vi "Seq Dialog Send LIN Message for inalfa SCU.vi"(8 "Segment Data":T3) -> (0 "Step Hisitory":string[](array[string]), 2 "Segment Data 2":T3)   [LabVIEW 2018]
uses:
  type defs/Sequence Info.ctl
  03.Inalfa LIN/LIN sequence for self SCU.ctl
  03.Inalfa LIN/LIN show Tags.ctl
  03.Inalfa LIN/LIN show messages.ctl
  <vilib>/Utility/error.llb/whitespace.ctl
panel:
  in  "Description":string
  in  "Tx2 2":u8[](array[numeric]) caption="Tx" format="%02x"
  in  "Checksunshade 2":bool=TRUE
  in  "Checkgalss 2":bool=TRUE
  in  "Sunshade Position 2":u16
  in  "Glass Position 2":u16
  in  "Rx 2":u8[](array[numeric]) format="%02x"
  in  "Tx 2":u8[](array[numeric]) format="%02x"
  in  "Slide Cycles 3":u16
  in  "Vent Cycles 3":u16
  in  "Slide Cycles 2":u16
  in  "Vent Cycles 2":u16
  out "LIN show Tags":T1
  in  "Vent Cycles":u16
  in  "Slide Cycles":u16
  in  "String":string
  in  "Tx2":u8[][](array[numeric]) format="%02x"
  in  "Rx":u8[](array[numeric]) format="%02x"
  in  "Tx":u8[][](array[numeric]) format="%02x"
  in  "Position":u16
  in  "Glass Position":u16
  in  "Sunshade Position":u16
  in  "Checkgalss":bool=TRUE
  in  "Checksunshade":bool=TRUE
  in  "Choose Sequence":T2
  out "String 2":string="Send LIN Message for self SCU"
  in  "Save":bool
  in  "Cancel":bool
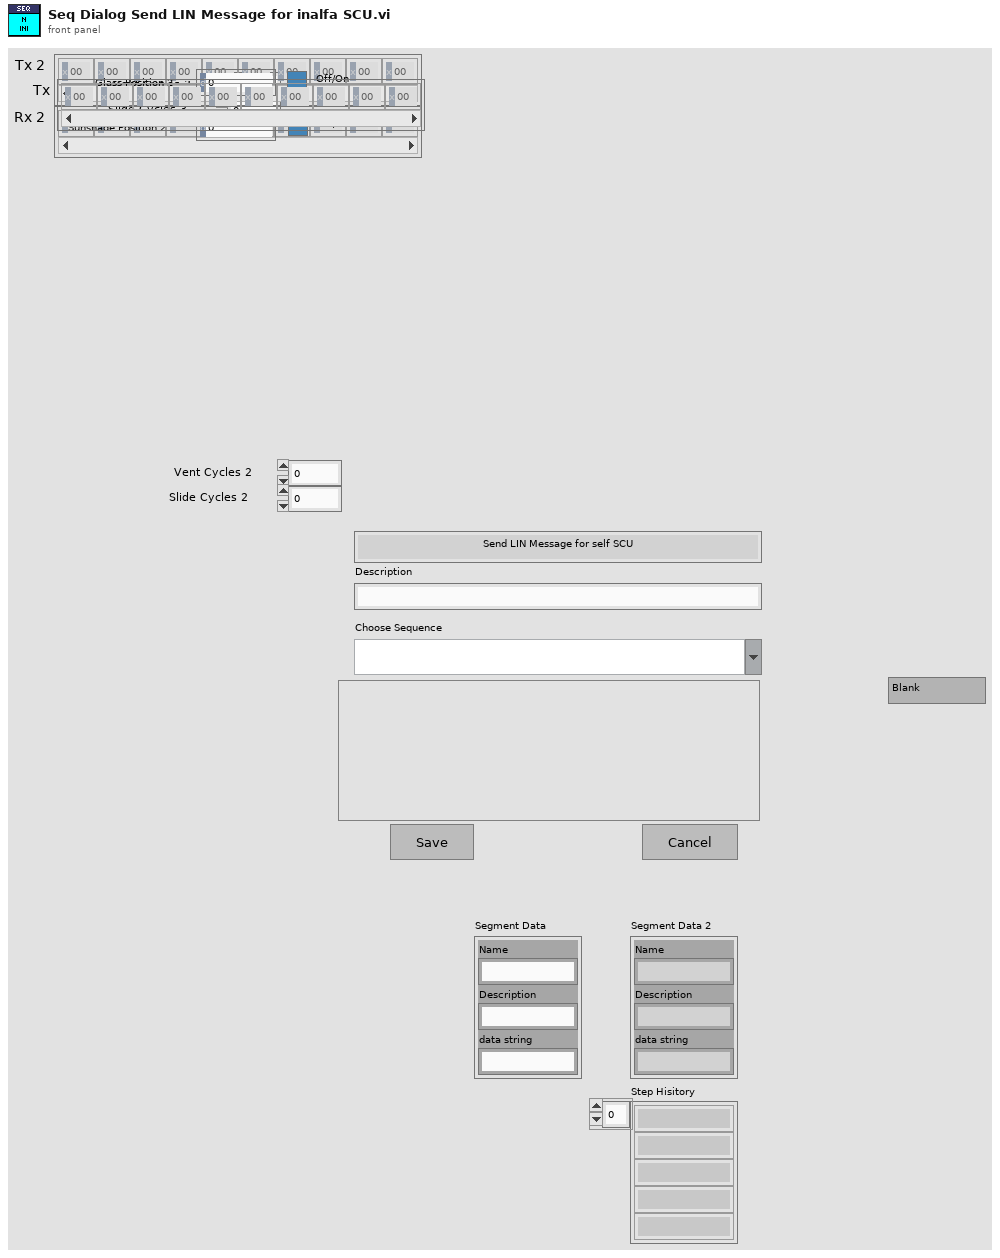
[diagram p1: front panel]
types:
  T1 = typedef "LIN show Tags.ctl" = enum32{"Blank", "Cycles", "String", "Tx", "Tx and Rx", "Go to position", "Check positions"}
  T2 = typedef "LIN sequence for self SCU.ctl" = string
  T3 = typedef "Sequence Info.ctl" = cluster{"Name":string, "Description":string, "data string":string}
  T4 = typedef "LIN show messages.ctl" = cluster{"Slide Cycles":u16, "Vent Cycles":u16, "String":string, "Tx Bytes":u8[][], "Rx Bytes":u8[], "Only Tx1 Bytes":u8[][], "Go to Position":u16, "Check Glass Position":u16, "Checkgalss":bool, "Check Sunshade Position":u16, "Checksunshade":bool}
  T5 = cluster{"LIN show messages":T4, "Segment Data":T3, "Old Data":string, "New Data":string}
  T6 = typedef "whitespace.ctl" = u16
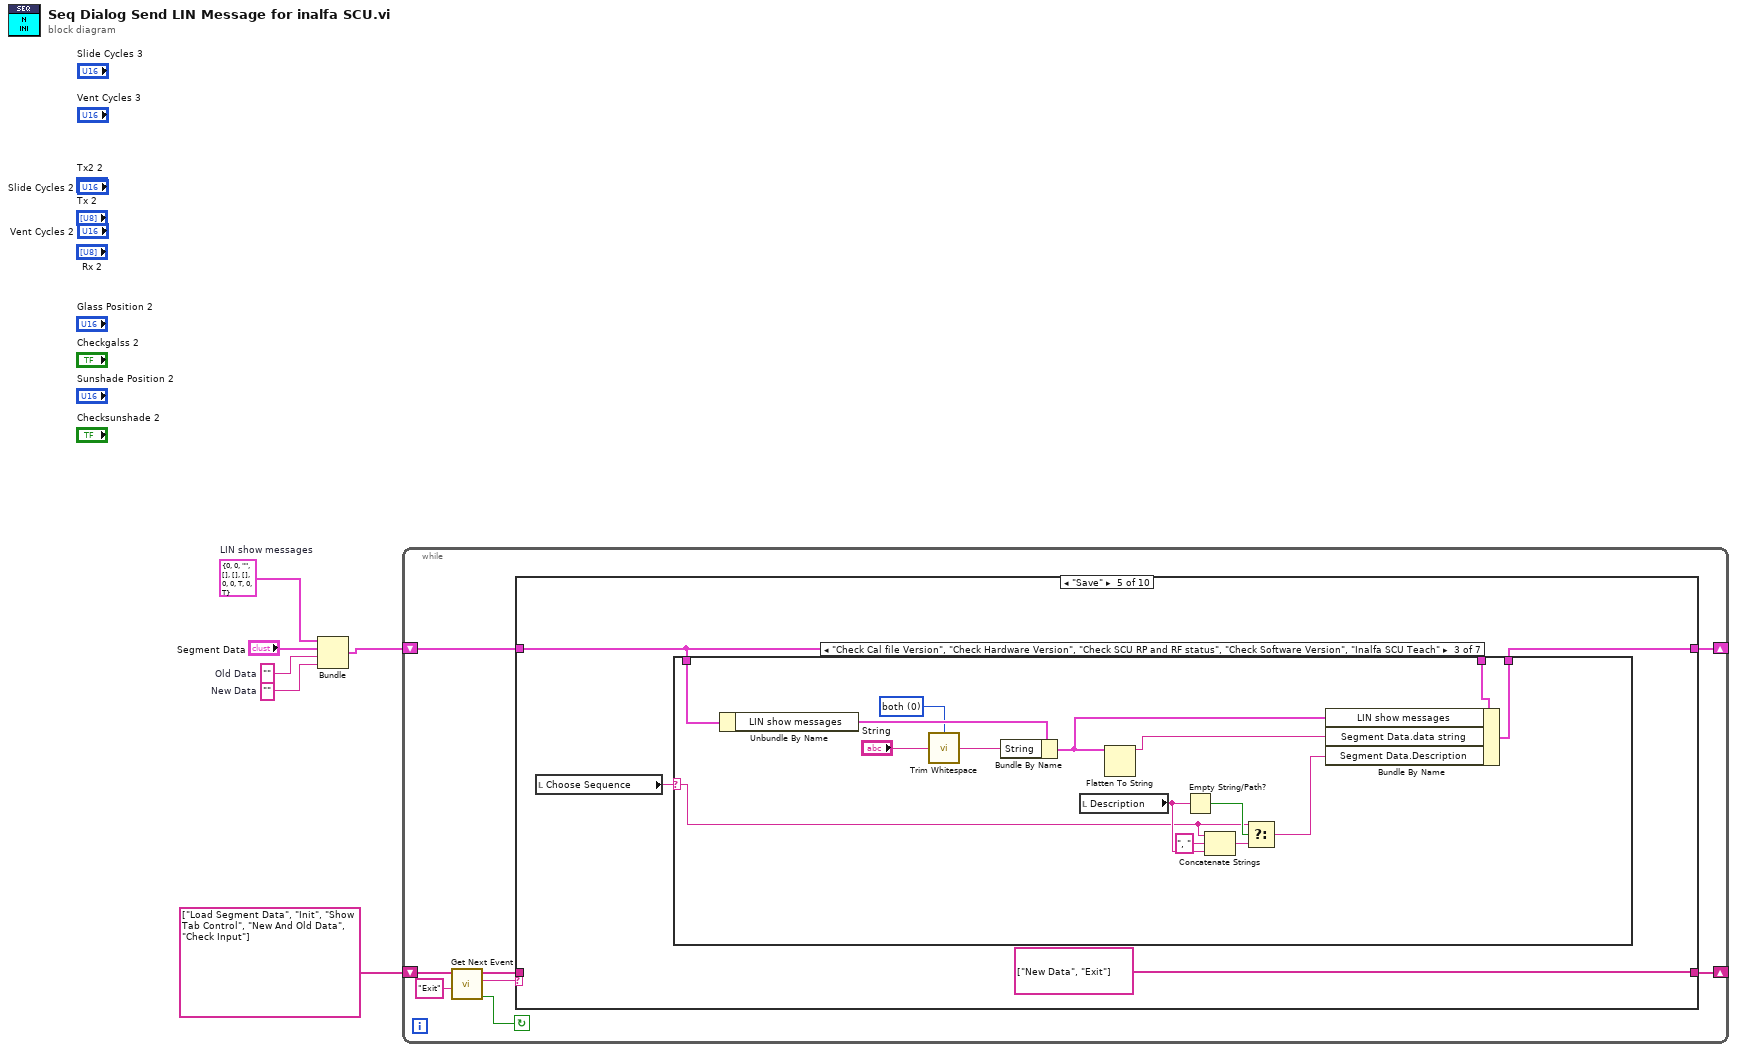
[diagram p0: block diagram]
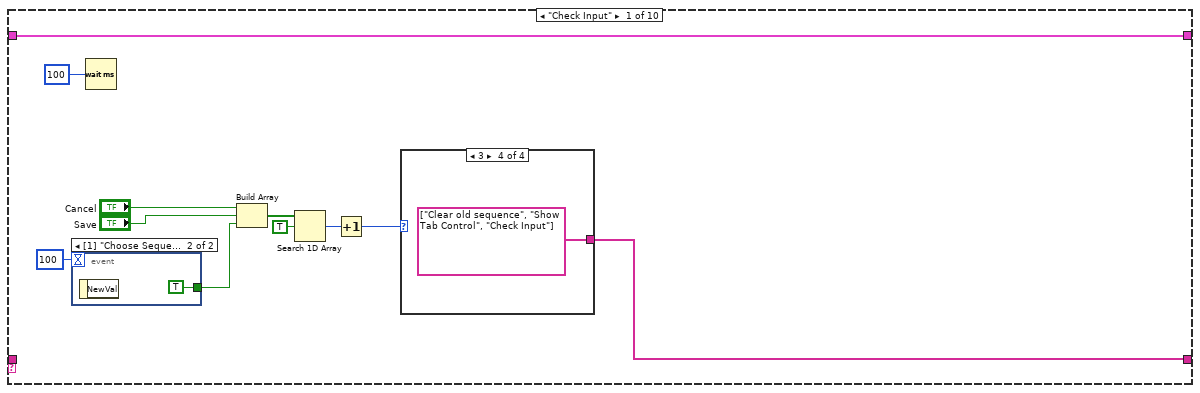
[diagram p2: hidden frame]
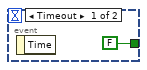
[diagram p3: hidden frame]
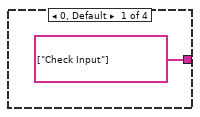
[diagram p4: hidden frame]
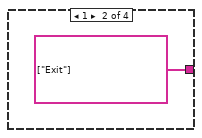
[diagram p5: hidden frame]
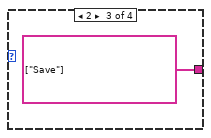
[diagram p6: hidden frame]
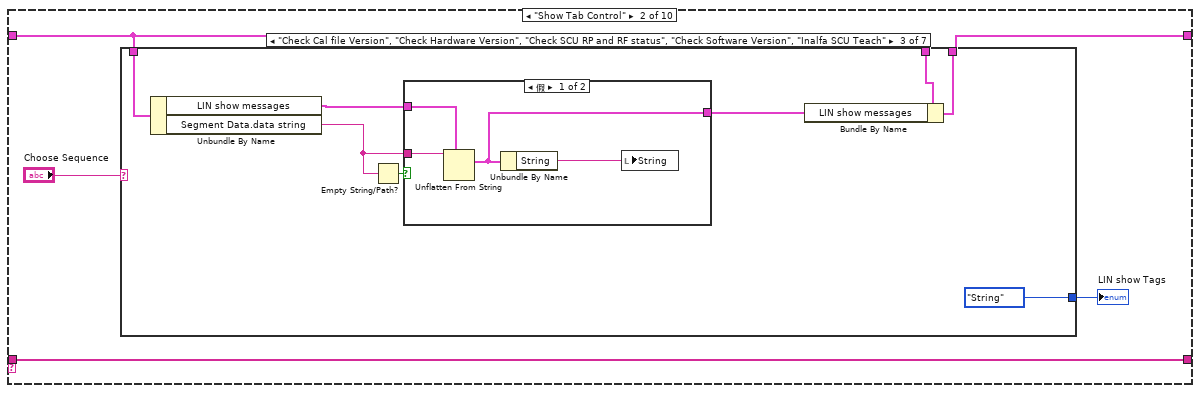
[diagram p7: hidden frame]
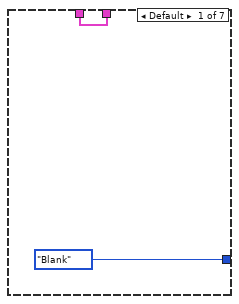
[diagram p8: hidden frame]
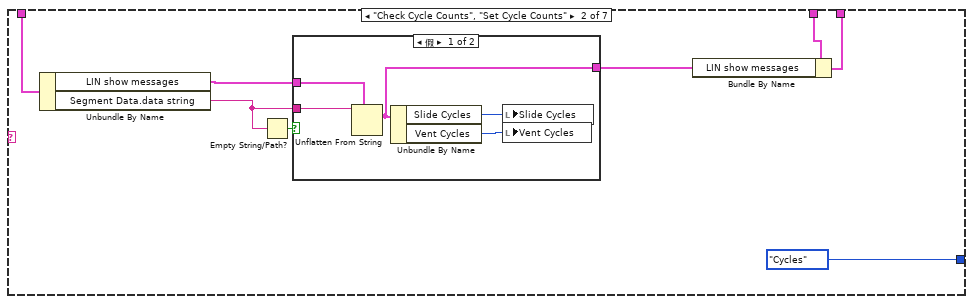
[diagram p9: hidden frame]
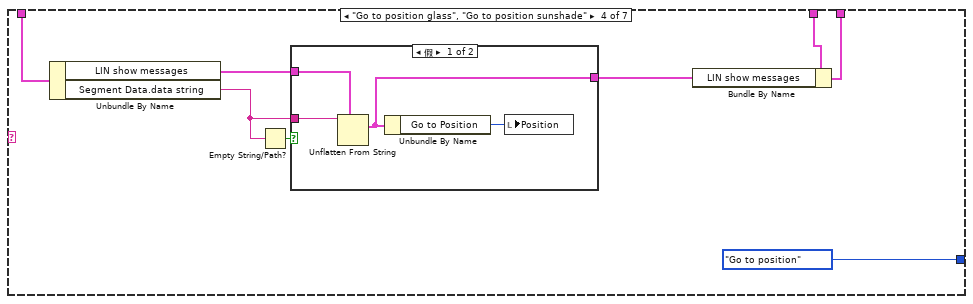
[diagram p12: hidden frame]
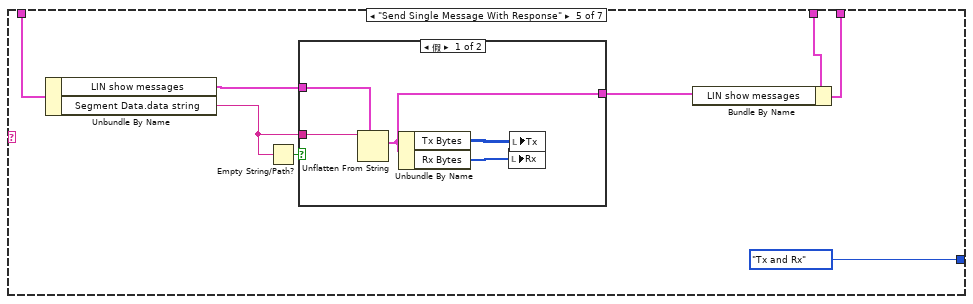
[diagram p14: hidden frame]
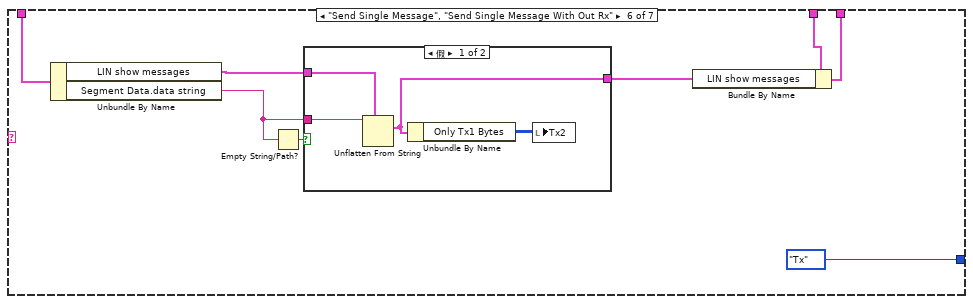
[diagram p16: hidden frame]
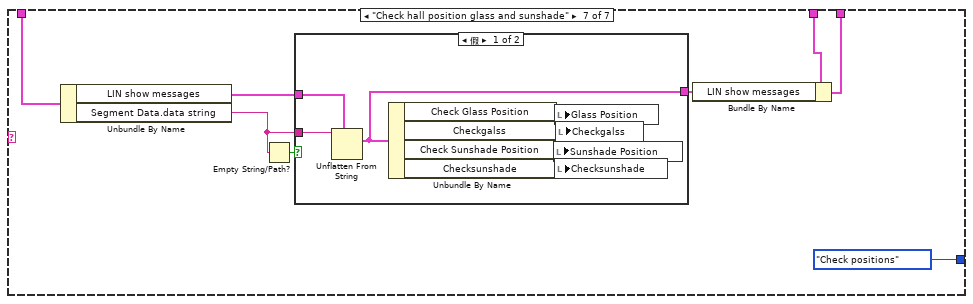
[diagram p18: hidden frame]
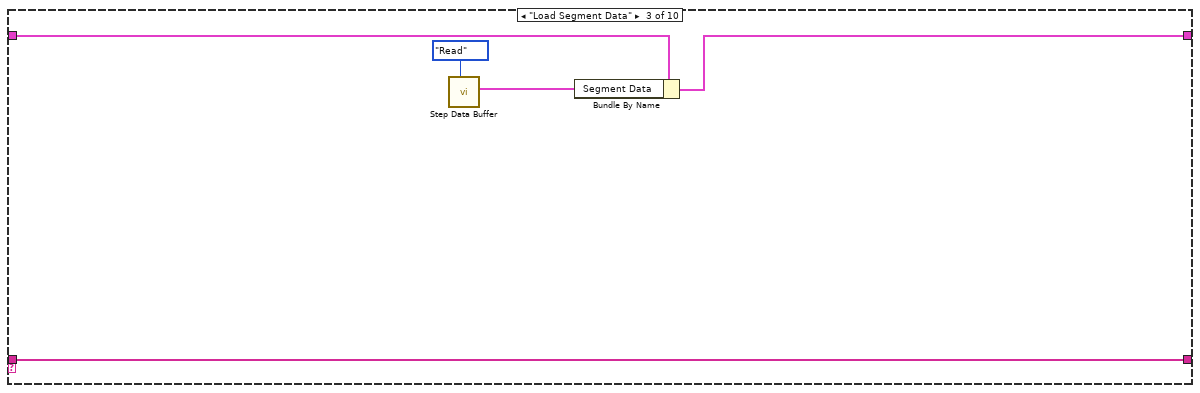
[diagram p20: hidden frame]
diagram:
  w3 = T4 {"Slide Cycles"=0, "Vent Cycles"=0, "String"="", "Tx Bytes"=[], "Rx Bytes"=[], "Only Tx1 Bytes"=[], "Go to Position"=0, "Check Glass Position"=0, "Checkgalss"=TRUE, "Check Sunshade Position"=0, "Checksunshade"=TRUE}  # LIN show messages
  w4 = ""  # New Data
  w5 = ""  # Old Data
  n1 = Bundle("LIN show messages"=w3, "Segment Data"="Segment Data", "Old Data"=w5, "New Data"=w4) -> (w2:T5)  [unwired: 1 in]
  n2 = while {
    shift-right: [w12] -> _
    shift-left: string[] ["Load Segment Data", "Init", "Show Tab Control", "New And Old Data", "Check Input"] ("Event queue out") -> [w11]
    shift-right: [w7] -> _
    shift-left: w2 -> [w8]
    stop <- w10 continue-if-true
    n3 = call "Get Next Event.vi"("Exit Event"="Exit", "event queue in"=w11) -> ("Condition (Exit:F)"=w10:bool, "next event"=w14:string, "event queue out"=w13:string[])  [unwired: 3 in]
    n4 = case shown="\"Save\"" w14 {
      selector: w14 -> [_ _ _ _ _ _ w245 _ _ _]
      tunnel: w13 -> [_ w36 w126 w131 _ w242 _ w255 w259 w368]
      tunnel: [w19 w36 w126 w131 string[] ["New Data", "Exit"] ("Event queue out") w242 string[] ["Exit"] ("event queue out") w255 w259 w368] -> w12
      tunnel: w8 -> [w24 w32 w123 w130 w134 w238 w243 w253 w258 w367]
      tunnel: [w24 w33 w122 w129 w133 w238 w243 w253 w257 w366] -> w7
      frame "Check Input" {
        n5 = event shown="[1] \"Choose Sequence\": 值改变" {
          selector: _ -> [_ _]
          dyn-events: _ -> [_ _]
          timeout: 100 -> [_ _]
          tunnel: [FALSE ("element") TRUE ("element")] -> w15
          event Timeout {
            n6 = event-data() -> ()  [unwired: 1 in, 1 out]
          }
          event Value Change {
            n7 = event-data() -> ()  [unwired: 1 in, 1 out]
          }
        }
        n8 = Wait (ms)(milliseconds to wait=u32 100) -> ()  [unwired: 1 out]
        n9 = Build Array("Cancel", "Save", w15) -> (w21:bool[])
        n10 = Search 1D Array(1D array=w21, element=TRUE) -> (index of element=w22:i32)  [unwired: 1 in]
        n11 = Increment(x=w22) -> (x+1=w23:i32)
        n12 = case shown="3" w23 {
          tunnel: [string[] ["Check Input"] ("Events to Insert") string[] ["Exit"] ("Events to Insert") string[] ["Save"] ("Events to Insert") string[] ["Clear old sequence", "Show Tab Control", "Check Input"] ("Events to Insert")] -> w19
          frame 0, Default {
          }
          frame 1 {
          }
          frame 2 {
          }
          frame 3 {
          }
        }
      }
      frame "Show Tab Control" {
        n13 = case shown="\"Check Cal file Version\", \"Check Hardware Version\", \"Check SCU RP and RF status\", \"Check Software Version\", \"Inalfa SCU Teach\"" "Choose Sequence" {
          tunnel: [LIN_show_Tags."Blank" ("LIN show Tags") LIN_show_Tags."Cycles" ("LIN show Tags") LIN_show_Tags."String" ("LIN show Tags") LIN_show_Tags."Go to position" ("LIN show Tags") LIN_show_Tags."Tx and Rx" ("LIN show Tags") LIN_show_Tags."Tx" ("LIN show Tags") LIN_show_Tags."Check positions" ("LIN show Tags")] -> w34
          tunnel: w32 -> [_ w43 w54 w67 w79 w95 w110]
          tunnel: w32 -> [w37 w41 w56 w69 w82 w94 w109]
          tunnel: [w37 w40 w55 w68 w81 w93 w108] -> w33
          frame Default {
          }
          frame "Check Cycle Counts", "Set Cycle Counts" {
            n14 = Unbundle By Name(w43) -> ("LIN show messages"=w42:T4, "Segment Data.data string"=w45:string)
            n15 = Empty String/Path?(string/path=w45) -> (empty?=w44:bool)
            n16 = case shown="假" w44 {
              tunnel: w45 -> [w51 _]
              tunnel: w42 -> [w48 w52]
              tunnel: [w47 w52] -> w39
              frame False {
                n17 = Unflatten From String(type=w48, binary string=w51) -> (value=w47:T4)  [unwired: 3 in, 2 out]
                n18 = Unbundle By Name(w47) -> ("Slide Cycles"=w50:u16, "Vent Cycles"=w49:u16)
                n19 = local write "Slide Cycles"(w50) -> ()
                n20 = local write "Vent Cycles"(w49) -> ()
              }
              frame True {
              }
            }
            n21 = Bundle By Name(cluster=w41, "LIN show messages"=w39) -> (w40:T5)
          }
          frame "Check Cal file Version", "Check Hardware Version", "Check SCU RP and RF status", "Check Software Version", "Inalfa SCU Teach" {
            n22 = Unbundle By Name(w54) -> ("LIN show messages"=w59:T4, "Segment Data.data string"=w57:string)
            n23 = Empty String/Path?(string/path=w57) -> (empty?=w58:bool)
            n24 = case shown="假" w58 {
              tunnel: w57 -> [w63 _]
              tunnel: w59 -> [w64 w65]
              tunnel: [w61 w65] -> w53
              frame False {
                n25 = Unflatten From String(type=w64, binary string=w63) -> (value=w61:T4)  [unwired: 3 in, 2 out]
                n26 = Unbundle By Name(w61) -> ("String"=w62:string)
                n27 = local write "String"(w62) -> ()
              }
              frame True {
              }
            }
            n28 = Bundle By Name(cluster=w56, "LIN show messages"=w53) -> (w55:T5)
          }
          frame "Go to position glass", "Go to position sunshade" {
            n29 = Unbundle By Name(w67) -> ("LIN show messages"=w72:T4, "Segment Data.data string"=w70:string)
            n30 = Empty String/Path?(string/path=w70) -> (empty?=w71:bool)
            n31 = case shown="假" w71 {
              tunnel: w70 -> [w75 _]
              tunnel: w72 -> [w77 w78]
              tunnel: [w76 w78] -> w66
              frame False {
                n32 = Unflatten From String(type=w77, binary string=w75) -> (value=w76:T4)  [unwired: 3 in, 2 out]
                n33 = Unbundle By Name(w76) -> ("Go to Position"=w74:u16)
                n34 = local write "Position"(w74) -> ()
              }
              frame True {
              }
            }
            n35 = Bundle By Name(cluster=w69, "LIN show messages"=w66) -> (w68:T5)
          }
          frame "Send Single Message With Response" {
            n36 = Unbundle By Name(w79) -> ("LIN show messages"=w85:T4, "Segment Data.data string"=w83:string)
            n37 = Empty String/Path?(string/path=w83) -> (empty?=w84:bool)
            n38 = case shown="假" w84 {
              tunnel: w83 -> [w91 _]
              tunnel: w85 -> [w88 w92]
              tunnel: [w87 w92] -> w80
              frame False {
                n39 = Unflatten From String(type=w88, binary string=w91) -> (value=w87:T4)  [unwired: 3 in, 2 out]
                n40 = Unbundle By Name(w87) -> ("Tx Bytes"=w90:u8[][], "Rx Bytes"=w89:u8[])
                n41 = local write "Rx"(w89) -> ()
                n42 = local write "Tx"(w90) -> ()
              }
              frame True {
              }
            }
            n43 = Bundle By Name(cluster=w82, "LIN show messages"=w80) -> (w81:T5)
          }
          frame "Send Single Message", "Send Single Message With Out Rx" {
            n44 = Unbundle By Name(w95) -> ("LIN show messages"=w99:T4, "Segment Data.data string"=w97:string)
            n45 = Empty String/Path?(string/path=w97) -> (empty?=w98:bool)
            n46 = case shown="假" w98 {
              tunnel: w97 -> [w104 _]
              tunnel: w99 -> [w103 w105]
              tunnel: [w102 w105] -> w96
              frame False {
                n47 = Unflatten From String(type=w103, binary string=w104) -> (value=w102:T4)  [unwired: 3 in, 2 out]
                n48 = Unbundle By Name(w102) -> ("Only Tx1 Bytes"=w101:u8[][])
                n49 = local write "Tx2"(w101) -> ()
              }
              frame True {
              }
            }
            n50 = Bundle By Name(cluster=w94, "LIN show messages"=w96) -> (w93:T5)
          }
          frame "Check hall position glass and sunshade" {
            n51 = Unbundle By Name(w110) -> ("LIN show messages"=w107:T4, "Segment Data.data string"=w111:string)
            n52 = Empty String/Path?(string/path=w111) -> (empty?=w112:bool)
            n53 = case shown="假" w112 {
              tunnel: w111 -> [w120 _]
              tunnel: [w114 w121] -> w106
              tunnel: w107 -> [w115 w121]
              frame False {
                n54 = Unflatten From String(type=w115, binary string=w120) -> (value=w114:T4)  [unwired: 3 in, 2 out]
                n55 = Unbundle By Name(w114) -> ("Check Glass Position"=w119:u16, "Checkgalss"=w118:bool, "Check Sunshade Position"=w117:u16, "Checksunshade"=w116:bool)
                n56 = local write "Sunshade Position"(w117) -> ()
                n57 = local write "Glass Position"(w119) -> ()
                n58 = local write "Checksunshade"(w116) -> ()
                n59 = local write "Checkgalss"(w118) -> ()
              }
              frame True {
              }
            }
            n60 = Bundle By Name(cluster=w109, "LIN show messages"=w106) -> (w108:T5)
          }
        }
        "LIN show Tags" <- w34
      }
      frame "Load Segment Data" {
        n61 = call "Step Data Buffer.vi"("Mode"=enum16{"Init", "Read", "Write"}."Read") -> ("Segment Data Out"=w125:T3)  [unwired: 6 in, 4 out]
        n62 = Bundle By Name(cluster=w123, "Segment Data"=w125) -> (w122:T5)
      }
      frame "Clear old sequence" {
        w127 = ""
        n63 = Bundle By Name(cluster=w130, "Segment Data.data string"=w127, "LIN show messages"=T4 {"Slide Cycles"=0, "Vent Cycles"=0, "String"="", "Tx Bytes"=[], "Rx Bytes"=[], "Only Tx1 Bytes"=[], "Go to Position"=0, "Check Glass Position"=0, "Checkgalss"=TRUE, "Check Sunshade Position"=0, "Checksunshade"=TRUE}) -> (w129:T5)
        n64 = local write "Description"(w127) -> ()
      }
      frame "Save" {
        n65 = local read "Choose Sequence"() -> (w132:T2)
        n66 = case shown="\"Check Cal file Version\", \"Check Hardware Version\", \"Check SCU RP and RF status\", \"Check Software Version\", \"Inalfa SCU Teach\"" w132 {
          selector: w132 -> [w136 w150 w168 w180 w192 w207 w220]
          tunnel: w134 -> [_ w162 w177 w190 w204 w217 w233]
          tunnel: w134 -> [w139 w161 w175 w189 w203 w215 w231]
          tunnel: [w138 w160 w174 w188 w202 w214 w230] -> w133
          frame Default {
            n67 = Empty String/Path?(string/path=w136) -> (empty?=w137:bool)
            n68 = case shown="假" w137 {
              tunnel: w139 -> [w147 w148]
              tunnel: [w146 w148] -> w138
              tunnel: w136 -> [w141 _]
              frame False {
                n69 = local read "Description"() -> (w144:string)
                n70 = Empty String/Path?(string/path=w144) -> (empty?=w143:bool)
                n71 = Concatenate Strings(w141, ", ", w144) -> (w142:string)
                n72 = Select(t=w141, s=w143, f=w142) -> (s? t:f=w140:string)
                n73 = Bundle By Name(cluster=w147, "Segment Data.Description"=w140) -> (w146:T5)
              }
              frame True {
              }
            }
          }
          frame "Check Cycle Counts", "Set Cycle Counts" {
            n74 = Unbundle By Name(w162) -> ("LIN show messages"=w159:T4)
            n75 = Bundle By Name(cluster=w159, "Slide Cycles"="Slide Cycles", "Vent Cycles"="Vent Cycles") -> (w157:T4)
            n76 = Flatten To String(anything=w157) -> (data string=w158:string)  [unwired: 3 in, 2 out]
            n77 = Empty String/Path?(string/path="Description") -> (empty?=w153:bool)
            n78 = Concatenate Strings(w150, ", ", "Description") -> (w152:string)
            n79 = Select(t=w150, s=w153, f=w152) -> (s? t:f=w149:string)
            n80 = Bundle By Name(cluster=w161, "LIN show messages"=w157, "Segment Data.data string"=w158, "Segment Data.Description"=w149) -> (w160:T5)
          }
          frame "Check Cal file Version", "Check Hardware Version", "Check SCU RP and RF status", "Check Software Version", "Inalfa SCU Teach" {
            w163 = T6 0 items=["both", "start of string", "end of string"] ("location (both)")
            n81 = Unbundle By Name(w177) -> ("LIN show messages"=w176:T4)
            n82 = call <vilib>:"Trim Whitespace.vi"("string"="String", "location (both)"=w163) -> ("trimmed string"=w164:string)
            n83 = Bundle By Name(cluster=w176, "String"=w164) -> (w165:T4)
            n84 = local read "Description"() -> (w171:string)
            n85 = Flatten To String(anything=w165) -> (data string=w166:string)  [unwired: 3 in, 2 out]
            n86 = Empty String/Path?(string/path=w171) -> (empty?=w170:bool)
            n87 = Concatenate Strings(w168, ", ", w171) -> (w169:string)
            n88 = Select(t=w168, s=w170, f=w169) -> (s? t:f=w167:string)
            n89 = Bundle By Name(cluster=w175, "LIN show messages"=w165, "Segment Data.data string"=w166, "Segment Data.Description"=w167) -> (w174:T5)
          }
          frame "Go to position glass", "Go to position sunshade" {
            n90 = Unbundle By Name(w190) -> ("LIN show messages"=w187:T4)
            n91 = Bundle By Name(cluster=w187, "Go to Position"="Position") -> (w178:T4)
            n92 = Flatten To String(anything=w178) -> (data string=w186:string)  [unwired: 3 in, 2 out]
            n93 = local read "Description"() -> (w183:string)
            n94 = Empty String/Path?(string/path=w183) -> (empty?=w182:bool)
            n95 = Concatenate Strings(w180, ", ", w183) -> (w181:string)
            n96 = Select(t=w180, s=w182, f=w181) -> (s? t:f=w179:string)
            n97 = Bundle By Name(cluster=w189, "LIN show messages"=w178, "Segment Data.data string"=w186, "Segment Data.Description"=w179) -> (w188:T5)
          }
          frame "Send Single Message With Response" {
            n98 = Unbundle By Name(w204) -> ("LIN show messages"=w201:T4)
            n99 = Bundle By Name(cluster=w201, "Tx Bytes"="Tx", "Rx Bytes"="Rx") -> (w198:T4)
            n100 = local read "Description"() -> (w195:string)
            n101 = Flatten To String(anything=w198) -> (data string=w197:string)  [unwired: 3 in, 2 out]
            n102 = Empty String/Path?(string/path=w195) -> (empty?=w194:bool)
            n103 = Concatenate Strings(w192, ", ", w195) -> (w193:string)
            n104 = Select(t=w192, s=w194, f=w193) -> (s? t:f=w191:string)
            n105 = Bundle By Name(cluster=w203, "LIN show messages"=w198, "Segment Data.data string"=w197, "Segment Data.Description"=w191) -> (w202:T5)
          }
          frame "Send Single Message", "Send Single Message With Out Rx" {
            n106 = Unbundle By Name(w217) -> ("LIN show messages"=w216:T4)
            n107 = Bundle By Name(cluster=w216, "Only Tx1 Bytes"="Tx2") -> (w213:T4)
            n108 = local read "Description"() -> (w210:string)
            n109 = Flatten To String(anything=w213) -> (data string=w212:string)  [unwired: 3 in, 2 out]
            n110 = Empty String/Path?(string/path=w210) -> (empty?=w209:bool)
            n111 = Concatenate Strings(w207, ", ", w210) -> (w208:string)
            n112 = Select(t=w207, s=w209, f=w208) -> (s? t:f=w206:string)
            n113 = Bundle By Name(cluster=w215, "LIN show messages"=w213, "Segment Data.data string"=w212, "Segment Data.Description"=w206) -> (w214:T5)
          }
          frame "Check hall position glass and sunshade" {
            n114 = Unbundle By Name(w233) -> ("LIN show messages"=w232:T4)
            n115 = Bundle By Name(cluster=w232, "Check Glass Position"="Glass Position", "Checkgalss"="Checkgalss", "Check Sunshade Position"="Sunshade Position", "Checksunshade"="Checksunshade") -> (w229:T4)
            n116 = local read "Description"() -> (w222:string)
            n117 = Flatten To String(anything=w229) -> (data string=w228:string)  [unwired: 3 in, 2 out]
            n118 = Empty String/Path?(string/path=w222) -> (empty?=w221:bool)
            n119 = Concatenate Strings(w220, ", ", w222) -> (w219:string)
            n120 = Select(t=w220, s=w221, f=w219) -> (s? t:f=w218:string)
            n121 = Bundle By Name(cluster=w231, "LIN show messages"=w229, "Segment Data.data string"=w228, "Segment Data.Description"=w218) -> (w230:T5)
          }
        }
      }
      frame "Exit" {
        n122 = Unbundle By Name(w238) -> ("Segment Data"=w236:T3, "Segment Data.Name"=w240:string, "Old Data"=w239:string, "New Data"=w241:string, "Segment Data.Description"=w234:string)
        "Segment Data 2" <- w236
        n123 = Build Array(w240, w239, w241, w234) -> (w235:string[])
        "Step Hisitory" <- w235
        n124 = call "Step Data Buffer.vi"("Mode"=enum16{"Init", "Read", "Write"}."Write", "Step Hisitory In"=w235, "Segment Data In"=w236) -> ()  [unwired: 4 in, 5 out]
      }
      frame "Error", Default {
        n125 = Concatenate Strings("Entered Error State - Intended State was - " ("string"), w245) -> (w247:string)
        n126 = One Button Dialog(message=w247) -> ()  [unwired: 1 in, 1 out]
      }
      frame "Init" {
        n127 = Unbundle By Name(w253) -> ("Segment Data.Description"=w251:string, "Segment Data.Name"=→"String 2":string)
        n128 = property on="Cancel" class="Bool (严格)"("Value"=FALSE ("Cancel")) -> ()  [unwired: 2 in, 2 out]
        n129 = Match Pattern(string=w251, regular expression=", ") -> (before substring=w248:string, after substring=w249:string)  [unwired: 1 in, 2 out]
        n130 = local write "Choose Sequence"(w248) -> ()
        n131 = local write "Description"(w249) -> ()
      }
      frame "New And Old Data" {
        n132 = local read "Choose Sequence"() -> (w256:T2)
        n133 = case shown="\"Set Cycle Counts\"" w256 {
          tunnel: w258 -> [_ w266 w279 w287 w298 w327 w348]
          tunnel: w258 -> [w260 w263 w281 w289 w300 w326 w343]
          tunnel: [w260 w262 w280 w288 w299 w325 w342] -> w257
          frame Default {
          }
          frame "Set Cycle Counts" {
            n134 = Unbundle By Name(w266) -> ("LIN show messages.Slide Cycles"=w265:u16, "LIN show messages.Vent Cycles"=w264:u16, "Segment Data.data string"=w268:string)
            n135 = Empty String/Path?(string/path=w268) -> (empty?=w267:bool)
            n136 = case shown="假" w267 {
              tunnel: w265 -> [w271 _]
              tunnel: w264 -> [w270 _]
              tunnel: [w269 "NA"] -> w261
              frame False {
                n137 = Format Into String(w271) -> (resulting string=w273:string)  [unwired: 3 in, 1 out]
                n138 = Format Into String(w270) -> (resulting string=w272:string)  [unwired: 3 in, 1 out]
                n139 = Concatenate Strings("Vent Cycles :" ("string"), w273, ", Slide Cycles :" ("string"), w272) -> (w269:string)
              }
              frame True {
              }
            }
            n140 = Bundle By Name(cluster=w263, "New Data"=w261, "Old Data"=w261) -> (w262:T5)
          }
          frame "Check Cal file Version", "Check Hardware Version", "Check Software Version" {
            n141 = Unbundle By Name(w279) -> ("LIN show messages.String"=w283:string, "Segment Data.data string"=w277:string)
            n142 = Empty String/Path?(string/path=w277) -> (empty?=w282:bool)
            n143 = case shown="假" w282 {
              tunnel: w283 -> [w284 _]
              tunnel: [w284 "NA"] -> w278
              frame False {
              }
              frame True {
              }
            }
            n144 = Bundle By Name(cluster=w281, "LIN show messages.String"=w278) -> (w280:T5)
          }
          frame "Go to position glass", "Go to position sunshade" {
            n145 = Unbundle By Name(w287) -> ("LIN show messages.Go to Position"=w292:u16, "Segment Data.data string"=w290:string)
            n146 = Empty String/Path?(string/path=w290) -> (empty?=w291:bool)
            n147 = case shown="假" w291 {
              tunnel: w292 -> [w294 _]
              tunnel: [w293 "NA"] -> w286
              frame False {
                n148 = Format Into String(initial string="Go To Position :" ("string"), w294) -> (resulting string=w293:string)  [unwired: 2 in, 1 out]
              }
              frame True {
              }
            }
            n149 = Bundle By Name(cluster=w289, "New Data"=w286, "Old Data"=w286) -> (w288:T5)
          }
          frame "Send Single Message With Response" {
            n150 = Unbundle By Name(w298) -> ("LIN show messages.Tx Bytes"=w301:u8[][], "LIN show messages.Rx Bytes"=w304:u8[], "Segment Data.data string"=w302:string)
            n151 = Empty String/Path?(string/path=w302) -> (empty?=w303:bool)
            n152 = case shown="假" w303 {
              tunnel: w304 -> [w306 _]
              tunnel: w301 -> [w307 _]
              tunnel: [w305 "NA"] -> w297
              frame False {
                n153 = Array To Spreadsheet String(delimiter (Tab)=" ", array=w307, 3:"%2x" ("format string")) -> (spreadsheet string=w318:string)
                n154 = Array To Spreadsheet String(delimiter (Tab)=" ", array=w306, 3:"%2x" ("format string")) -> (spreadsheet string=w320:string)
                n155 = call <vilib>:"Space Constant.vi"() -> ("String"=w317:string)
                n156 = call <vilib>:"Space Constant.vi"() -> ("String"=w321:string)
                n157 = Search and Replace String(input string=w318, search string="\r\n", replace string=w317) -> (result string=w319:string)  [unwired: 5 in, 3 out]
                n158 = Search and Replace String(input string=w320, search string="\r\n", replace string=w321) -> (result string=w322:string)  [unwired: 5 in, 3 out]
                n159 = Concatenate Strings("Data Bytes :" ("string"), "TX: " ("string"), w319, ", RX: " ("string"), w322) -> (w305:string)
              }
              frame True {
              }
            }
            n160 = Bundle By Name(cluster=w300, "New Data"=w297, "Old Data"=w297) -> (w299:T5)
          }
          frame "Send Single Message", "Send Single Message With Out Rx" {
            n161 = Unbundle By Name(w327) -> ("LIN show messages.Only Tx1 Bytes"=w330:u8[][], "Segment Data.data string"=w328:string)
            n162 = Empty String/Path?(string/path=w328) -> (empty?=w329:bool)
            n163 = case shown="假" w329 {
              tunnel: w330 -> [w331 _]
              tunnel: [w332 "NA"] -> w324
              frame False {
                n164 = Array To Spreadsheet String(delimiter (Tab)=" ", array=w331, 3:"%2x" ("format string")) -> (spreadsheet string=w338:string)
                n165 = call <vilib>:"Space Constant.vi"() -> ("String"=w339:string)
                n166 = Search and Replace String(input string=w338, search string="\r\n", replace string=w339) -> (result string=w337:string)  [unwired: 5 in, 3 out]
                n167 = Concatenate Strings("Data Bytes :" ("string"), w337) -> (w332:string)
              }
              frame True {
              }
            }
            n168 = Bundle By Name(cluster=w326, "New Data"=w324, "Old Data"=w324) -> (w325:T5)
          }
          frame "Check hall position glass and sunshade" {
            n169 = Unbundle By Name(w348) -> ("LIN show messages.Check Glass Position"=w347:u16, "LIN show messages.Checkgalss"=w346:bool, "LIN show messages.Check Sunshade Position"=w345:u16, "LIN show messages.Checksunshade"=w344:bool, "Segment Data.data string"=w349:string)
            n170 = Empty String/Path?(string/path=w349) -> (empty?=w350:bool)
            n171 = case shown="假" w350 {
              tunnel: w349 -> [_ _]
              tunnel: w347 -> [w358 _]
              tunnel: w346 -> [w359 _]
              tunnel: w345 -> [w357 _]
              tunnel: w344 -> [w356 _]
              tunnel: [w351 "NA"] -> w341
              frame False {
                n172 = Format Into String(initial string="Glass Position :" ("string"), w358) -> (resulting string=w355:string)  [unwired: 2 in, 1 out]
                n173 = Format Into String(initial string=", was Checked :" ("string"), w359) -> (resulting string=w354:string)  [unwired: 2 in, 1 out]
                n174 = Format Into String(initial string=", Sunshade Position :" ("string"), w357) -> (resulting string=w353:string)  [unwired: 2 in, 1 out]
                n175 = Format Into String(initial string=", was Checked :" ("string"), w356) -> (resulting string=w352:string)  [unwired: 2 in, 1 out]
                n176 = Concatenate Strings(w355, w354, w353, w352) -> (w351:string)
              }
              frame True {
              }
            }
            n177 = Bundle By Name(cluster=w343, "New Data"=w341, "Old Data"=w341) -> (w342:T5)
          }
        }
      }
      frame "New Data" {
        n178 = local read "Choose Sequence"() -> (w365:T2)
        n179 = case shown="\"Check Cal file Version\", \"Check Hardware Version\", \"Check Software Version\"" w365 {
          tunnel: w367 -> [_ w379 w381 w386 w406 w421 w438]
          tunnel: w367 -> [w369 w376 w383 w388 w408 w420 w433]
          tunnel: [w369 w375 w382 w387 w407 w419 w432] -> w366
          frame Default {
          }
          frame "Set Cycle Counts" {
            n180 = Unbundle By Name(w379) -> ("LIN show messages.Slide Cycles"=w378:u16, "LIN show messages.Vent Cycles"=w377:u16)
            n181 = Format Into String(w378) -> (resulting string=w371:string)  [unwired: 3 in, 1 out]
            n182 = Format Into String(w377) -> (resulting string=w370:string)  [unwired: 3 in, 1 out]
            n183 = Concatenate Strings("Vent Cycles :" ("string"), w371, ", Slide Cycles :" ("string"), w370) -> (w374:string)
            n184 = Bundle By Name(cluster=w376, "New Data"=w374) -> (w375:T5)
          }
          frame "Check Cal file Version", "Check Hardware Version", "Check Software Version" {
            n185 = Unbundle By Name(w381) -> ("LIN show messages.String"=w380:string)
            n186 = Bundle By Name(cluster=w383, "LIN show messages.String"=w380) -> (w382:T5)
          }
          frame "Go to position glass", "Go to position sunshade" {
            n187 = Unbundle By Name(w386) -> ("LIN show messages.Go to Position"=w389:u16)
            n188 = Format Into String(initial string="Go To Position :" ("string"), w389) -> (resulting string=w385:string)  [unwired: 2 in, 1 out]
            n189 = Bundle By Name(cluster=w388, "New Data"=w385) -> (w387:T5)
          }
          frame "Send Single Message With Response" {
            n190 = Unbundle By Name(w406) -> ("LIN show messages.Tx Bytes"=w409:u8[][], "LIN show messages.Rx Bytes"=w410:u8[])
            n191 = Array To Spreadsheet String(delimiter (Tab)=" ", array=w409, 3:"%2x" ("format string")) -> (spreadsheet string=w400:string)
            n192 = Array To Spreadsheet String(delimiter (Tab)=" ", array=w410, 3:"%2x" ("format string")) -> (spreadsheet string=w402:string)
            n193 = call <vilib>:"Space Constant.vi"() -> ("String"=w399:string)
            n194 = call <vilib>:"Space Constant.vi"() -> ("String"=w403:string)
            n195 = Search and Replace String(input string=w400, search string="\r\n", replace string=w399) -> (result string=w401:string)  [unwired: 5 in, 3 out]
            n196 = Search and Replace String(input string=w402, search string="\r\n", replace string=w403) -> (result string=w404:string)  [unwired: 5 in, 3 out]
            n197 = Concatenate Strings("Data Bytes :" ("string"), "TX: " ("string"), w401, ", RX: " ("string"), w404) -> (w405:string)
            n198 = Bundle By Name(cluster=w408, "New Data"=w405) -> (w407:T5)
          }
          frame "Send Single Message", "Send Single Message With Out Rx" {
            n199 = Unbundle By Name(w421) -> ("LIN show messages.Only Tx1 Bytes"=w422:u8[][])
            n200 = Array To Spreadsheet String(delimiter (Tab)=" ", array=w422, 3:"%2x" ("format string")) -> (spreadsheet string=w416:string)
            n201 = call <vilib>:"Space Constant.vi"() -> ("String"=w417:string)
            n202 = Search and Replace String(input string=w416, search string="\r\n", replace string=w417) -> (result string=w415:string)  [unwired: 5 in, 3 out]
            n203 = Concatenate Strings("Data Bytes :" ("string"), w415) -> (w418:string)
            n204 = Bundle By Name(cluster=w420, "New Data"=w418, "Old Data"=w418) -> (w419:T5)
          }
          frame "Check hall position glass and sunshade" {
            n205 = Unbundle By Name(w438) -> ("LIN show messages.Check Glass Position"=w437:u16, "LIN show messages.Checkgalss"=w436:bool, "LIN show messages.Check Sunshade Position"=w435:u16, "LIN show messages.Checksunshade"=w434:bool)
            n206 = Format Into String(initial string="Glass Position :" ("string"), w437) -> (resulting string=w426:string)  [unwired: 2 in, 1 out]
            n207 = Format Into String(initial string=", was Checked :" ("string"), w436) -> (resulting string=w425:string)  [unwired: 2 in, 1 out]
            n208 = Format Into String(initial string=", Sunshade Position :" ("string"), w435) -> (resulting string=w424:string)  [unwired: 2 in, 1 out]
            n209 = Format Into String(initial string=", was Checked :" ("string"), w434) -> (resulting string=w423:string)  [unwired: 2 in, 1 out]
            n210 = Concatenate Strings(w426, w425, w424, w423) -> (w431:string)
            n211 = Bundle By Name(cluster=w433, "New Data"=w431) -> (w432:T5)
          }
        }
      }
    }
  }
